vi "Find Top Panel.vi"(10 "Scroll":i32, 11 "All Panels":refnum<class "ArrayPanel.lvclass">[](array[class])) -> (2 "Start":i32, 3 "Panels":refnum<class "ArrayPanel.lvclass">[](array[class]))   [LabVIEW 2020, in "OOPanel.lvlib" / "ArrayManager.lvclass"]
uses:
  ArrayManager.lvclass
  ArrayManager.lvclass/ArrayManager.ctl
  ArrayPanel/ArrayPanel.lvclass
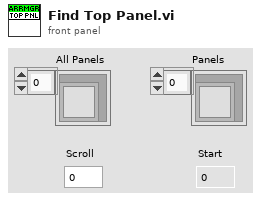
[diagram p1: front panel]
types:
  T1 = typedef "OOPanel.lvlib/Desired Size.ctl" = cluster{"Width":u32, "Height":u32}
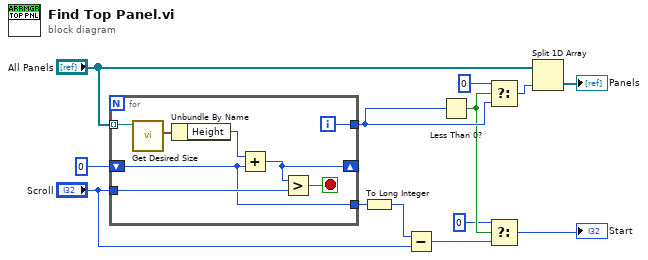
[diagram p0: block diagram]
diagram:
  n1 = for {
    tunnel: "Scroll" -> [w18]
    tunnel: "All Panels" -> [w21] mode=indexing
    shift-right: [w16] -> _
    shift-left: u32 0 -> [w14]
    tunnel: [w15] -> w12
    tunnel: [w14] -> w6
    i -> [w15]
    stop <- w17 stop-if-true
    n2 = call-dynamic "Get Desired Size.vi"("ArrayPanel in"=w21) -> ("Desired Size"=w20:T1)  [unwired: 8 in, 2 out]
    n3 = Unbundle By Name(w20) -> ("Height"=w19:u32)
    n4 = Add(x=w19, y=w14) -> (x+y=w16:u32)
    n5 = Greater?(x=w16, y=w18) -> (0:w17:bool)
  }
  n6 = To Long Integer(number=w6) -> (32bit integer=w1:i32)
  n7 = Subtract(x=w1, y="Scroll") -> (x-y=w5:i32)
  n8 = Less Than 0?(x=w12) -> (x < 0?=w4:bool)
  n9 = Select(t=0, s=w4, f=w12) -> (s? t:f=w9:i32)
  n10 = Select(t=u32 0, s=w4, f=w5) -> (s? t:f=→"Start":u32)
  n11 = Split 1D Array(array="All Panels", index=w9) -> (second subarray=→"Panels":refnum<class "ArrayPanel.lvclass">[])  [unwired: 1 out]
